vi "EvaluateOpStateExit.vi"(8 "error in (no error)":errorcluster, 9 "data flow":T2, 10 "config":T1, 11 "Qbus in":refnum<class "Qbus.lvclass">) -> (0 "error out":errorcluster, 2 "config out":T1)   [LabVIEW 2017, in "EmsaDataEventCreator.lvlib"]
uses:
  <vilib>/addons/InsightCM/Devices/Shared/Emsa/EmsaDataEventCreator/EmsaDataEventCreator.lvlib
  <vilib>/addons/InsightCM/Devices/Shared/Common/DataFlow/controls/Data.ctl
  <vilib>/addons/InsightCM/Utilities/DataAccessors/controls/wfmSGL_DVR.ctl
  <vilib>/addons/PointValueMap/controls/PointMap.ctl
  <vilib>/addons/InsightCM/Devices/Shared/Common/DataFlow/controls/Type.ctl
  <vilib>/addons/Qbus/Qbus.lvclass
  <vilib>/addons/InsightCM/Devices/Shared/Emsa/EmsaDataEventCreator/controls/config.ctl
  <vilib>/addons/InsightCM/Devices/Shared/Emsa/EmsaDataEventCreator/controls/SweepParams.ctl
  <vilib>/addons/InsightCM/Devices/Shared/Common/DataEventCreator/controls/Reason.ctl
  <vilib>/addons/InsightCM/Devices/Shared/Emsa/EmsaDataEventCreator/controls/DataEventConfig.ctl
  <vilib>/addons/PointValueMap/subVIs/Point_Read_string.vi
  <vilib>/addons/PointValueMap/PointValueMap.lvlib
  <vilib>/addons/InsightCM/Devices/Shared/Common/DataEventCreator/DataEventCreator.lvlib
  <vilib>/addons/InsightCM/Devices/Shared/Common/DataFlow/DataFlow.lvlib
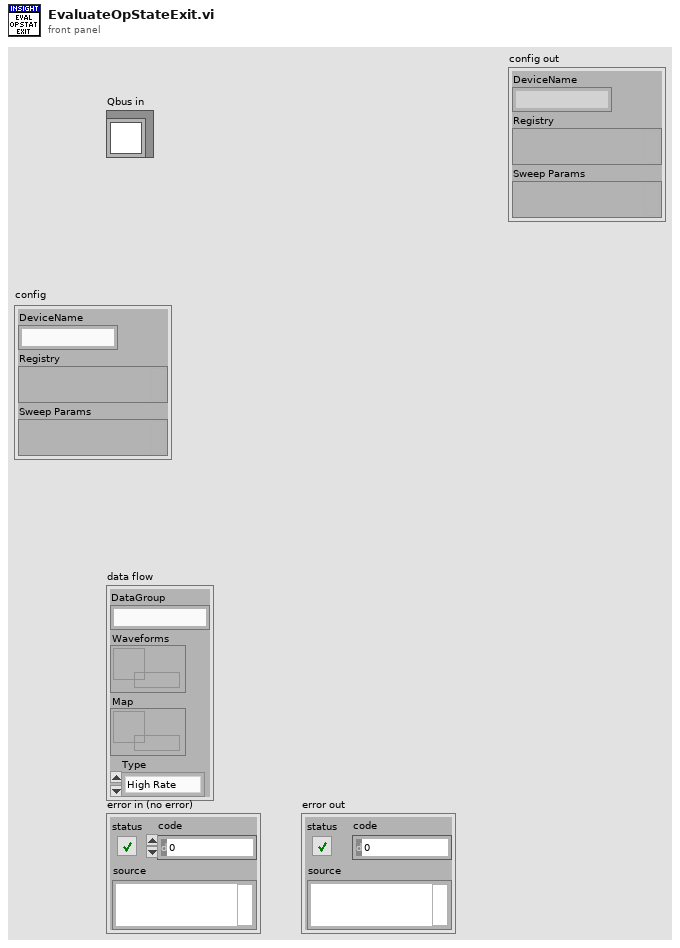
[diagram p1: front panel]
types:
  T1 = typedef "EmsaDataEventCreator.lvlib/config.ctl" = cluster{"DeviceName":string, "Registry":variant, "Sweep Params":variant}
  T2 = typedef "DataFlow.lvlib/Data.ctl" = cluster{"DataGroup":string, "Waveforms":T3, "Map":T4, "Type":T5}
  T3 = typedef "wfmSGL_DVR.ctl" = refnum<data-value>
  T4 = typedef "PointValueMap.lvlib/PointMap.ctl" = refnum<data-value>
  T5 = typedef "DataFlow.lvlib/Type.ctl" = enum16{"High Rate", "Low Rate", "Burst Mode"}
  T6 = typedef "DataEventCreator.lvlib/Reason.ctl" = enum16{"Periodic Event", "Delta EU Event", "Trend Event", "Alarm Event", "User Event", "Enter Operating State", "Exit Operating State", "Multiple Events", "Other"}
  T7 = typedef "EmsaDataEventCreator.lvlib/SweepParams.ctl" = cluster{"CollectOnEnter":bool, "CollectOnExit":bool}
  T8 = typedef "EmsaDataEventCreator.lvlib/DataEventConfig.ctl" = cluster{"OpState":string, "ExitOpState":bool, "Reason":string, "StreamId":string, "Map":T4, "DataSetIds":variant, "IncludeWaveforms":bool, "TrendPointsOnly":bool, "Sweep Params":T7}
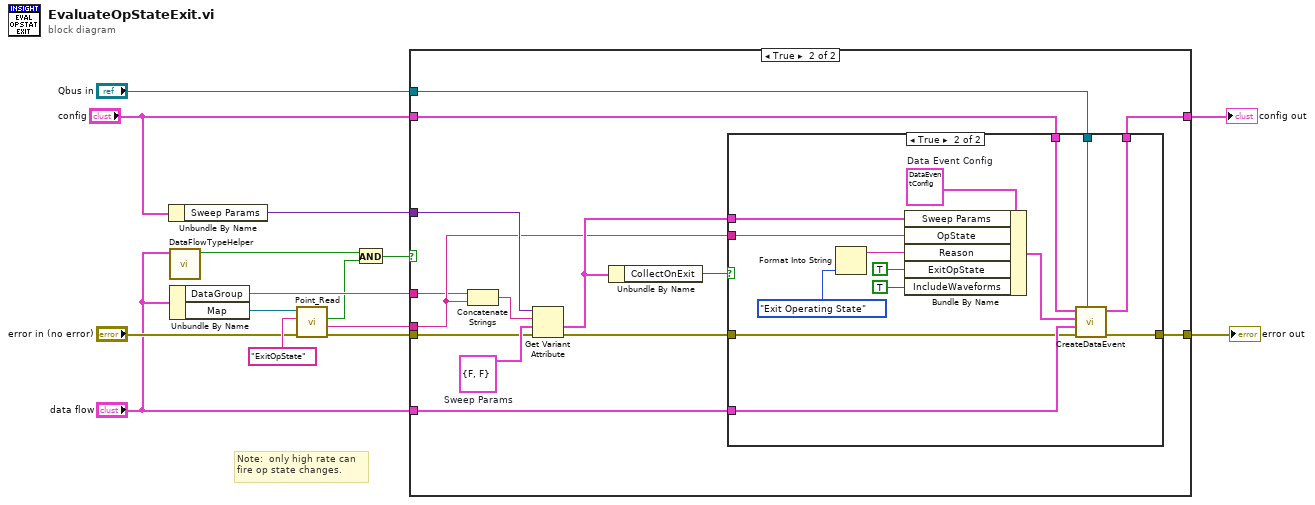
[diagram p0: block diagram]
diagram:
  # "Note:  only high rate can\nfire op state changes."
  n1 = Unbundle By Name("config") -> ("Sweep Params"=w8:variant)
  n2 = call <vilib>:"DataFlowTypeHelper.vi"("data"="data flow") -> ("high rate"=w2:bool)  [unwired: 8 in, 2 out]
  n3 = Unbundle By Name("data flow") -> ("DataGroup"=w10:string, "Map"=w15:T4)
  n4 = call-poly <vilib>:"Point_Read.vi"("Error In"="error in (no error)", "Tag"="ExitOpState", "Map"=w15) -> ("Error Out"=w12:errorcluster, "Value"=w11:string, "Found?"=w6:bool)  [unwired: 3 in, 3 out]
  n5 = And(x=w2, y=w6) -> (x .and. y?=w5:bool)
  n6 = case shown="True" w5 {
    tunnel: w12 -> [w16 w20]
    tunnel: w11 -> [_ w23]
    tunnel: w10 -> [_ w22]
    tunnel: w8 -> [_ w30]
    tunnel: "config" -> [w17 w18]
    tunnel: [w17 w28] -> w3
    tunnel: "data flow" -> [_ w27]
    tunnel: "Qbus in" -> [_ w26]
    tunnel: [w16 w25] -> w9
    frame False {
    }
    frame True {
      w21 = T7 {"CollectOnEnter"=FALSE, "CollectOnExit"=FALSE}  # Sweep Params
      n7 = Concatenate Strings(w22, w23) -> (w31:string)
      n8 = Get Variant Attribute(Variant=w30, name=w31, default value (empty Variant)=w21, error in=w20) -> (value=w29:T7, error out=w19:errorcluster)  [unwired: 2 out]
      n9 = Unbundle By Name(w29) -> ("CollectOnExit"=w24:bool)
      n10 = case shown="True" w24 {
        tunnel: w29 -> [_ w47]
        tunnel: [w33 w46] -> w28
        tunnel: w27 -> [_ w45]
        tunnel: w26 -> [_ w44]
        tunnel: [w32 w43] -> w25
        tunnel: w19 -> [w32 w42]
        tunnel: w18 -> [w33 w41]
        tunnel: w23 -> [_ w40]
        frame False {
        }
        frame True {
          w34 = T8 {"OpState"="", "ExitOpState"=FALSE, "Reason"="", "StreamId"="", "Map"=refnum, "DataSetIds"=variant, "IncludeWaveforms"=FALSE, "TrendPointsOnly"=FALSE, "Sweep Params"={"CollectOnEnter"=FALSE, "CollectOnExit"=FALSE}}  # Data Event Config
          n11 = Format Into String(Reason."Exit Operating State" ("Reason")) -> (resulting string=w36:string)  [unwired: 3 in, 1 out]
          n12 = Bundle By Name(cluster=w34, "Sweep Params"=w47, "OpState"=w40, "Reason"=w36, "ExitOpState"=TRUE, "IncludeWaveforms"=TRUE) -> (w39:T8)
          n13 = call <vilib>:"CreateDataEvent.vi"("Qbus"=w44, "error in (no error)"=w42, "data flow"=w45, "data event config"=w39, "config"=w41) -> ("error out"=w43:errorcluster, "config out"=w46:T1)  [unwired: 5 in]
        }
      }
    }
  }
  "error out" <- w9
  "config out" <- w3
